vi "Populate Variables in CMD.vi"(5 "Variant":variant, 6 "Error in":errorcluster caption="Error in (no error)", 9 "String might with variables":string) -> (0 "Error out":errorcluster, 3 "String out":string, 4 "Variant Out":variant)   [LabVIEW 2020, in "CSMStand(Lite).lvlib"]
uses:
  CSMStand(Lite).lvlib
  <userlib>/_NEVSTOP/Communicable State Machine(CSM)/_Shared/CSM Shared.lvlib
  <userlib>/_NEVSTOP/Communicable State Machine(CSM)/addons/INI-Static-Variable-Support/INI-Static-Variable-Support.lvlib
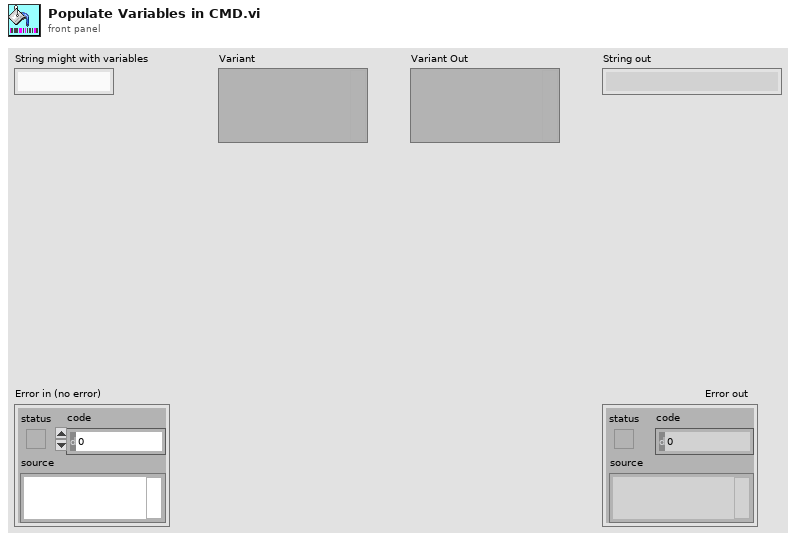
[diagram p1: front panel]
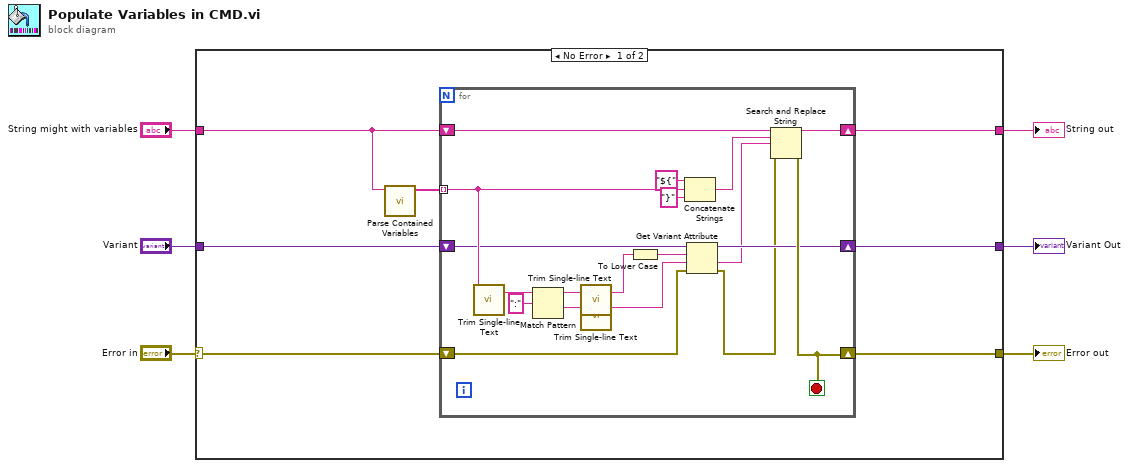
[diagram p0: block diagram]
diagram:
  n1 = case shown="No Error" "Error in" {
    selector: "Error in" -> [w7 w35]
    tunnel: [w13 w34] -> w6
    tunnel: "String might with variables" -> [w12 w34]
    tunnel: [w11 w35] -> w3
    tunnel: "Variant" -> [w10 w33]
    tunnel: [w9 w33] -> w1
    frame No Error {
      n2 = call <userlib>:"Parse Contained Variables.vi"("String"=w12) -> ("Contained Variables"=w8:string[])  [unwired: 10 in]
      n3 = for {
        tunnel: w8 -> [w30] mode=indexing
        shift-right: [w31] -> w13
        shift-left: w12 -> [w32]
        shift-right: [w29] -> w11
        shift-left: w7 -> [w28]
        shift-right: [w19] -> w9
        shift-left: w10 -> [w27]
        stop <- w29 stop-if-true
        n4 = call <userlib>:"Trim Single-line Text.vi"("single-line text"=w30) -> ("trimed text"=w22:string)  [unwired: 2 in]
        n5 = Match Pattern(string=w22, regular expression=":") -> (before substring=w25:string, after substring=w24:string)  [unwired: 1 in, 2 out]
        n6 = call <userlib>:"Trim Single-line Text.vi"("single-line text"=w25) -> ("trimed text"=w21:string)  [unwired: 2 in]
        n7 = call <userlib>:"Trim Single-line Text.vi"("single-line text"=w24) -> ("trimed text"=w23:string)  [unwired: 2 in]
        n8 = To Lower Case(string=w21) -> (all lower case string=w20:string)
        n9 = Concatenate Strings("${" ("regular expression"), w30, "}" ("regular expression")) -> (w14:string)
        n10 = Get Variant Attribute(Variant=w27, name=w20, default value (empty Variant)=w23, error in=w28) -> (duplicate Variant=w19:variant, value=w18:string, error out=w17:errorcluster)  [unwired: 1 out]
        n11 = Search and Replace String(input string=w32, search string=w14, replace string=w18, error in=w17) -> (result string=w31:string, error out=w29:errorcluster)  [unwired: 4 in, 2 out]
      }
    }
    frame Error {
    }
  }
  "String out" <- w6
  "Error out" <- w3
  "Variant Out" <- w1
